vi "Build Application.vi"(8 "error in (no error)":errorcluster, 11 "PostBuildSupport in":refnum<class "PostBuildSupport.lvclass">) -> (0 "error out":errorcluster, 3 "PostBuildSupport out":refnum<class "PostBuildSupport.lvclass">)   [LabVIEW 2016, in "PostBuildSupport.lvclass"]
uses:
  PostBuildSupport.lvclass
  <vilib>/AppBuilder/AB_API/common/AB_API Version Number.ctl
  PostBuildSupport.lvclass/PostBuildSupport.ctl
  <vilib>/AppBuilder/AB_API_Simple/Build (path).vi
  <vilib>/AppBuilder/AB_API/EXE/NI_AB_API_EXE.lvclass
  <vilib>/AppBuilder/AB_API_Simple/NI_App_Builder_API.lvlib
panel:
  out "error out 2":errorcluster
  in  "Project:Open":refnum<vi>
  out "GeneratedFiles":path[](array[path])
  in  "Build name":string
  in  "error in":errorcluster
  in  "Version number":T1
  in  "Cancel Button":bool
  out "Progress Bar":u8(slide) caption="Progress Bar..." scale=0.0..100.0
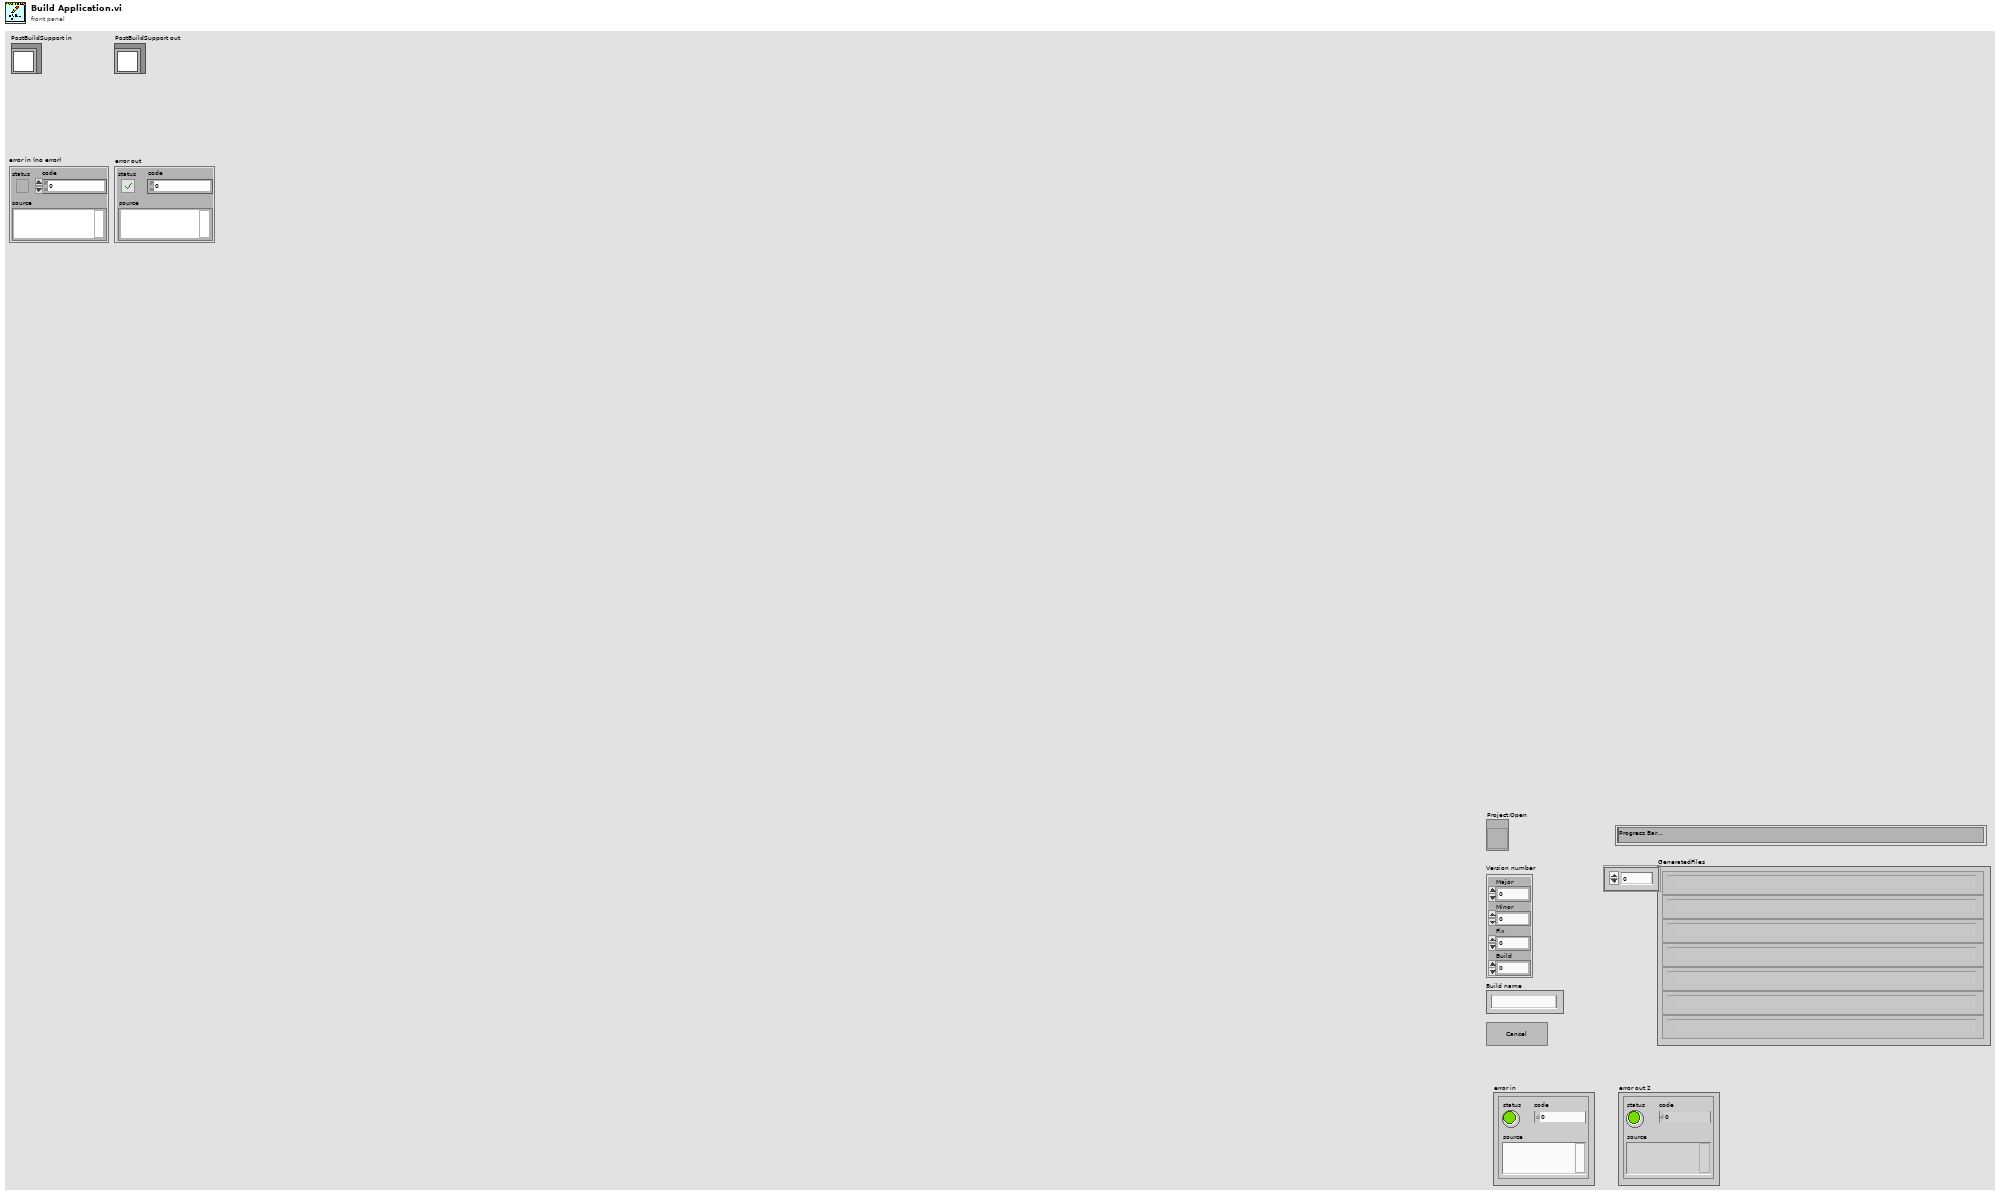
[diagram p1: front panel]
types:
  T1 = typedef "AB_API Version Number.ctl" = cluster{"Major":u16, "Minor":u16, "Fix":u16, "Build":u16}
  T2 = typedef "AB_API ProgressBar_Events.ctl" = cluster{"newJob":refnum<user-event>, "newItem":refnum<user-event>, "errorMsg":T3, "cancel":refnum<user-event>}
  T3 = typedef "AB_API ProgressBar_BuildError.ctl" = refnum<user-event>
  T4 = enum8{"Enabled", "Disabled", "Disabled and Grayed Out"}
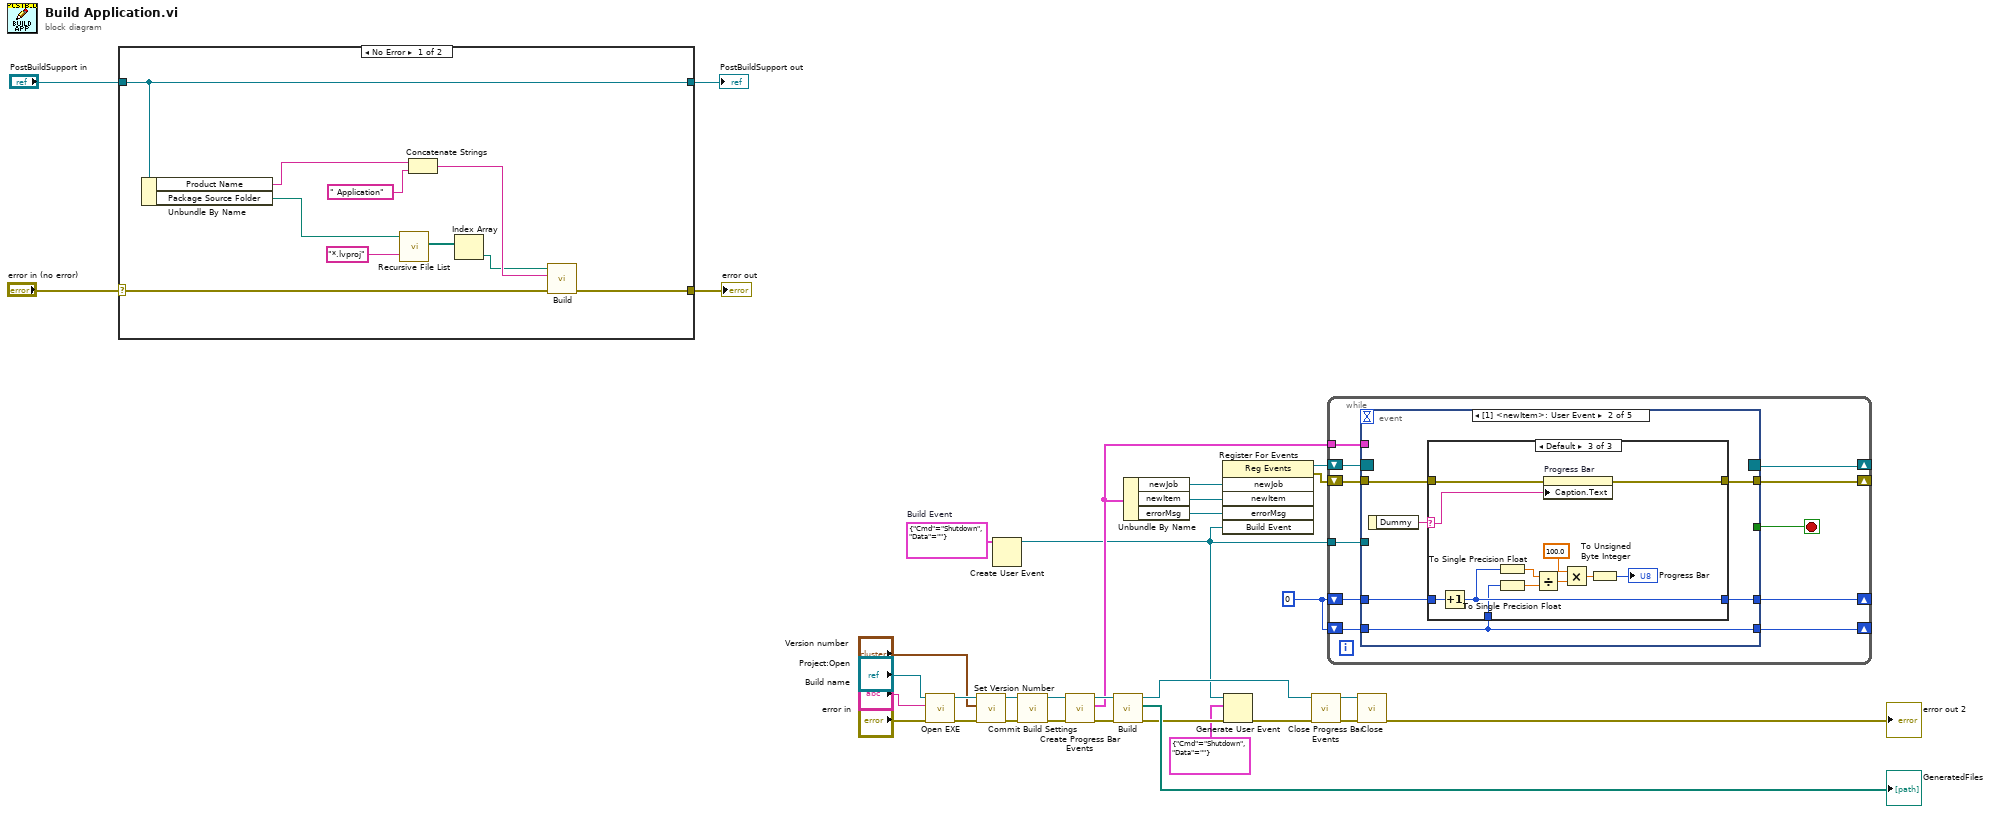
[diagram p0: block diagram]
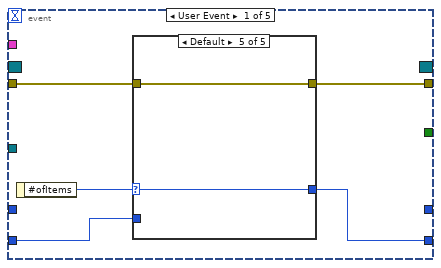
[diagram p2: hidden frame]
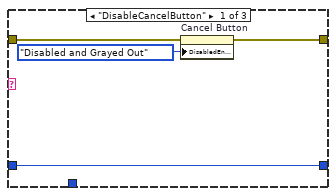
[diagram p7: hidden frame]
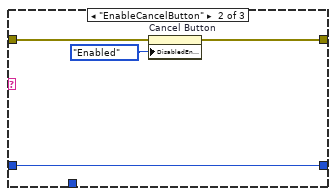
[diagram p8: hidden frame]
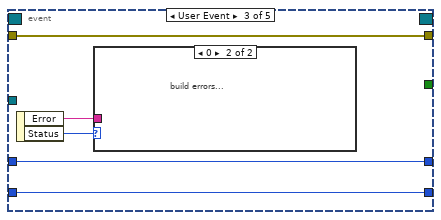
[diagram p9: hidden frame]
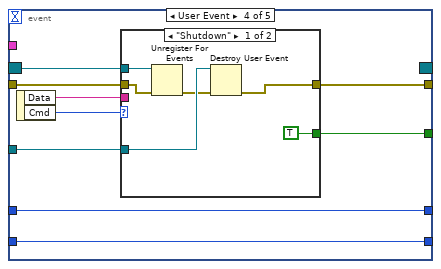
[diagram p11: hidden frame]
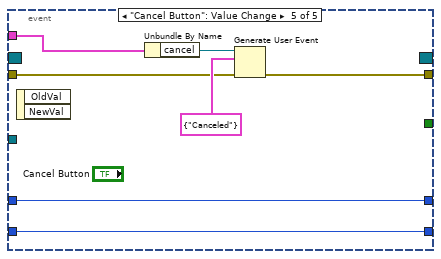
[diagram p13: hidden frame]
diagram:
  w7 = cluster{"Cmd":enum16{"Shutdown"}, "Data":string} {"Cmd"=enum."Shutdown", "Data"=""}  # Build Event
  w6 = 0 ("#ofItems")
  n1 = case shown="No Error" "error in (no error)" {
    selector: "error in (no error)" -> [w36 w45]
    tunnel: "PostBuildSupport in" -> [w35 w44]
    tunnel: [w37 w45] -> w31
    tunnel: [w35 w44] -> w30
    frame No Error {
      n2 = Unbundle By Name(w35) -> ("Product Name"=w39:string, "Package Source Folder"=w40:path)
      n3 = call <vilib>:"Recursive File List.vi"("pattern"="*.lvproj", "Folder Path"=w40) -> ("All Files in Dir"=w41:path[])  [unwired: 5 in, 4 out]
      n4 = Concatenate Strings(w39, " Application" ("Name of target (My Computer)")) -> (w38:string)
      n5 = Index Array(array=w41) -> (element=w34:path)  [unwired: 1 in]
      n6 = call-poly <vilib>:"Build.vi"("error in (no error)"=w36, "Name of build specification (if empty: build all)"=w38, "Path to project"=w34) -> ("error out"=w37:errorcluster)  [unwired: 7 in, 1 out]
    }
    frame Error {
    }
  }
  "error out" <- w31
  "PostBuildSupport out" <- w30
  n7 = call <vilib>:"Open EXE.vi"("error in (no error)"="error in", "Build specification name"="Build name", "Project Refnum"="Project:Open") -> ("error out"=w28:errorcluster, "EXE out"=w27:refnum<class "NI_AB_API_EXE.lvclass">)  [unwired: 7 in]
  n8 = call-dynamic "Set Version Number.vi"("error in (no error)"=w28, "Version number"="Version number", "EXE in"=w27) -> ("error out"=w26:errorcluster, "EXE out"=w20:refnum<class "NI_AB_API_EXE.lvclass">)  [unwired: 7 in]
  n9 = Create User Event(user event datatype=w7) -> (user event=w2:refnum<user-event>)  [unwired: 1 in, 1 out]
  n10 = call-dynamic "Commit Build Settings.vi"("error in (no error)"=w26, "EXE in"=w20) -> ("error out"=w14:errorcluster, "EXE out"=w19:refnum<class "NI_AB_API_EXE.lvclass">)  [unwired: 8 in]
  n11 = call-dynamic "Create Progress Bar Events.vi"("error in (no error)"=w14, "NI_AB_API_Build in"=w19) -> ("error out"=w13:errorcluster, "progressBarEvents"=w5:T2, "NI_AB_API_Build out"=w18:refnum<class "NI_AB_API_EXE.lvclass">)  [unwired: 7 in]
  n12 = call-dynamic <vilib>:"Build.vi"("error in (no error)"=w13, "EXE in"=w18) -> ("error out"=w4:errorcluster, "GeneratedFiles"=→"GeneratedFiles":path[], "EXE out"=w17:refnum<class "NI_AB_API_EXE.lvclass">)  [unwired: 6 in, 1 out]
  n13 = Unbundle By Name(w5) -> ("newJob"=w12:refnum<user-event>, "newItem"=w11:refnum<user-event>, "errorMsg"=w10:T3)
  n14 = register-events(w12, w11, w10, w2) -> (reference out=w9:refnum<event-registration>, error out=w8:errorcluster)  [unwired: 2 in]
  n15 = Generate User Event(user event=w2, event data cluster=cluster{"Cmd":enum16{"Shutdown"}, "Data":string} {"Cmd"=enum."Shutdown", "Data"=""} ("event data"), error in=w4) -> (error out=w3:errorcluster)  [unwired: 1 in, 1 out]
  n16 = call-dynamic "Close Progress Bar Events.vi"("error in (no error)"=w3, "NI_AB_API_Build in"=w17) -> ("error out"=w15:errorcluster, "NI_AB_API_Build out"=w16:refnum<class "NI_AB_API_EXE.lvclass">)  [unwired: 8 in]
  n17 = while {
    shift-right: [w56] -> _
    shift-left: w8 -> [w53]
    shift-right: [w55] -> _
    shift-left: w9 -> [w54]
    shift-right: [w51] -> _
    shift-left: w6 -> [w48]
    shift-right: [w50] -> _
    shift-left: w6 -> [w49]
    tunnel: w2 -> [w47]
    tunnel: w5 -> [w46]
    stop <- w52 stop-if-true
    n18 = event shown="[1] <newItem>: User Event" {
      selector: w54 -> [_ _ _ w107 _]
      dyn-events: [_ _ _ _ _] -> w55
      timeout: _ -> [_ _ _ _ _]
      tunnel: [w60 w73 w102 w106 w123] -> w56
      tunnel: w53 -> [w61 w72 w102 w105 w119]
      tunnel: [_ _ _ w109 _] -> w52
      tunnel: [w58 w75 w100 w110 w122] -> w51
      tunnel: [_ w76 w101 w111 w121] -> w50
      tunnel: w49 -> [_ w74 w101 w111 w121]
      tunnel: w48 -> [w57 w75 w100 w110 w122]
      tunnel: w47 -> [_ _ _ w103 _]
      tunnel: w46 -> [_ _ _ _ w120]
      event User Event {
        n19 = event-data() -> ("#ofItems"=w59:i32)  [unwired: 1 in]
        n20 = case shown="Default" w59 {
          selector: w59 -> [w63 w65 w67 _ w71]
          tunnel: w61 -> [w62 w64 w66 w69 w70]
          tunnel: [w62 w64 w66 w69 w70] -> w60
          tunnel: [w63 w65 w67 w68 w71] -> w58
          tunnel: w57 -> [_ _ _ w68 _]
          frame -1 {
            # "Canceled response"
          }
          frame -2 {
          }
          frame -3 {
          }
          frame -4 {
          }
          frame Default {
          }
        }
      }
      event User Event {
        n21 = event-data() -> ("Dummy"=w77:string)  [unwired: 1 in]
        n22 = case shown="Default" w77 {
          selector: w77 -> [_ _ w88]
          tunnel: w74 -> [w80 w84 w95]
          tunnel: [w80 w84 w94] -> w76
          tunnel: w75 -> [_ _ w93]
          tunnel: [w78 w82 w86] -> w73
          tunnel: w72 -> [w79 w83 w87]
          frame "DisableCancelButton" {
            n23 = property on="Cancel Button" class="Bool"(error in=w79, "DisabledEnum"=T4."Disabled and Grayed Out" ("Disabled")) -> (error out=w78:errorcluster)  [unwired: 1 in, 1 out]
          }
          frame "EnableCancelButton" {
            n24 = property on="Cancel Button" class="Bool"(error in=w83, "DisabledEnum"=T4."Enabled" ("Disabled")) -> (error out=w82:errorcluster)  [unwired: 1 in, 1 out]
          }
          frame Default {
            n25 = Increment(x=w95) -> (x+1=w94:i32)
            n26 = To Single Precision Float(number=w94) -> (single precision float=w91:sgl)
            n27 = To Single Precision Float(number=w93) -> (single precision float=w90:sgl)
            n28 = Divide(x=w91, y=w90) -> (x/y=w92:sgl)
            n29 = property on="Progress Bar" class="Slide (strict)"(error in=w87, "Caption.Text"=w88) -> (error out=w86:errorcluster)  [unwired: 1 in, 1 out]
            n30 = Multiply(x=sgl 100.0, y=w92) -> (x*y=w97:sgl)
            n31 = To Unsigned Byte Integer(number=w97) -> (unsigned 8bit integer=→"Progress Bar":u8)
          }
        }
      }
      event User Event {
        n32 = event-data() -> ("Error"=w98:string, "Status"=w99:i32)  [unwired: 1 in]
        n33 = case shown="0" w99 {
          tunnel: w98 -> [_ _]
          frame Default {
          }
          frame 0 {
            # "build errors..."
          }
        }
      }
      event User Event {
        n34 = event-data() -> ("Data"=w104:string, "Cmd"=w108:enum16{"Shutdown"})  [unwired: 1 in]
        n35 = case shown="\"Shutdown\"" w108 {
          tunnel: [TRUE _] -> w109
          tunnel: w107 -> [w116 _]
          tunnel: [w112 w118] -> w106
          tunnel: w105 -> [w115 w118]
          tunnel: w104 -> [_ _]
          tunnel: w103 -> [w114 _]
          frame "Shutdown" {
            n36 = Unregister For Events(event registration refnum=w116, error in=w115) -> (error out=w113:errorcluster)
            n37 = Destroy User Event(user event=w114, error in=w113) -> (error out=w112:errorcluster)
          }
          frame Default {
          }
        }
      }
      event "Cancel Button": Value Change {
        n38 = event-data() -> ()  [unwired: 1 in, 2 out]
        n39 = Unbundle By Name(w120) -> ("cancel"=w124:refnum<user-event>)
        n40 = Generate User Event(user event=w124, event data cluster=cluster{"Dummy":string} {"Dummy"="Canceled"} ("event data"), error in=w119) -> (error out=w123:errorcluster)  [unwired: 1 in, 1 out]
      }
    }
  }
  n41 = call-dynamic "Close.vi"("error in (no error)"=w15, "EXE in"=w16) -> ("error out"=→"error out 2":errorcluster)  [unwired: 9 in]
